vi "close.vi"(8 "error in (no error)":errorcluster, 11 "Instrument in":refnum<class "Lock-In Amplifier.lvclass">) -> (0 "error out":errorcluster)   [LabVIEW 2020, in "Lock-In Amplifier.lvclass"]
uses:
  Lock-In Amplifier.lvclass
  Abstract Instrument/Abstract Instrument.lvclass
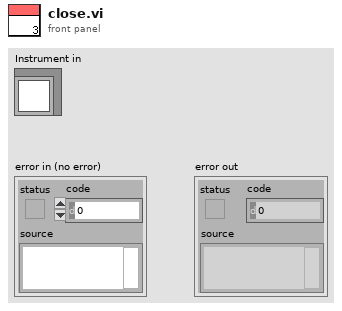
[diagram p1: front panel]
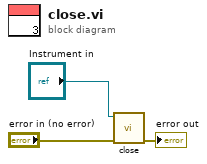
[diagram p0: block diagram]
diagram:
  n1 = call-parent "close.vi"("error in (no error)"="error in (no error)", "Instrument in"="Instrument in") -> ("error out"=→"error out":errorcluster)  [unwired: 9 in]
